vi "Global-velocity.vi"() -> ()   [LabVIEW 2020]
panel:
  out "global-velocity":dbl
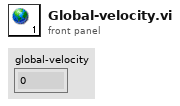
[diagram p1: front panel]
diagram:
